vi "GetAllPaths.vi"(0 "LocalName":string) -> (1 "Hard Path":path, 2 "Top Level":path, 3 "User Documents":path)   [LabVIEW 2012]
doc: "Gets the paths for LVROS, the servers, _BlankServer, and the Master Console"
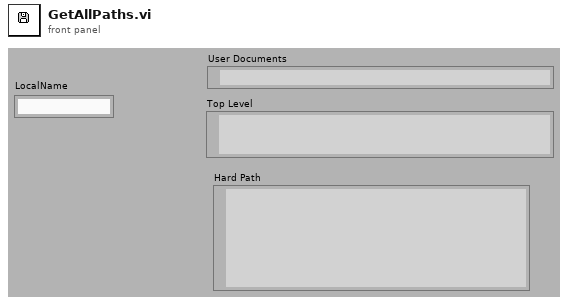
[diagram p1: front panel]
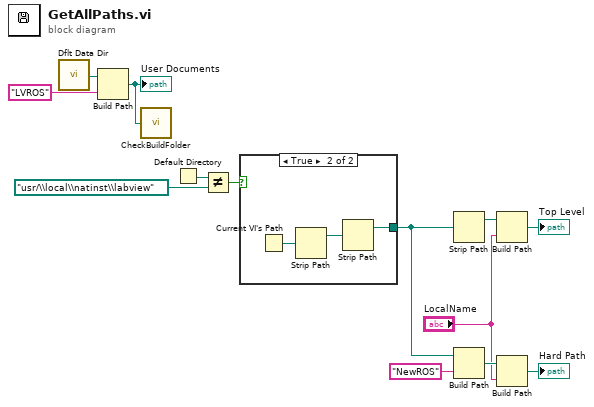
[diagram p0: block diagram]
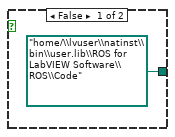
[diagram p2: hidden frame]
diagram:
  n1 = call <vilib>:"Dflt Data Dir.vi"() -> ("App:Default Data Directory"=w12:path)
  n2 = Build Path(base path=w12, name or relative path="LVROS") -> (appended path=w11:path)
  "User Documents" <- w11
  n3 = call <userlib>:"CheckBuildFolder.vi"("appended path"=w11) -> ()  [unwired: 1 in]
  n4 = Default Directory() -> (w2:path)
  n5 = Not Equal?(x=w2, y=path "/usr/\\local\\natinst\\labview") -> (x != y?=w3:bool)
  n6 = case shown="True" w3 {
    tunnel: [path "/home/\\lvuser\\natinst\\bin\\user.lib\\ROS for LabVIEW Software\\ROS\\Code" ("stripped path") w15] -> w7
    frame False {
    }
    frame True {
      n7 = Current VI's Path() -> (path=w17:path)
      n8 = Strip Path(path=w17) -> (stripped path=w16:path)  [unwired: 1 out]
      n9 = Strip Path(path=w16) -> (stripped path=w15:path)  [unwired: 1 out]
    }
  }
  n10 = Strip Path(path=w7) -> (stripped path=w6:path)  [unwired: 1 out]
  n11 = Build Path(base path=w7, name or relative path="NewROS") -> (appended path=w10:path)
  n12 = Build Path(base path=w6, name or relative path="LocalName") -> (appended path=→"Top Level":path)
  n13 = Build Path(base path=w10, name or relative path="LocalName") -> (appended path=→"Hard Path":path)
